vi "Find Safe Cell.vi"(0 "Cells":i32[](array[numeric]), 11 "error in (no error)":errorcluster) -> (4 "Safe Cells":i32[](array[numeric]), 6 "# of Safe Cells":i32, 15 "error out":errorcluster)   [LabVIEW 2014]
uses:
  Dragon Tamers.lvlib
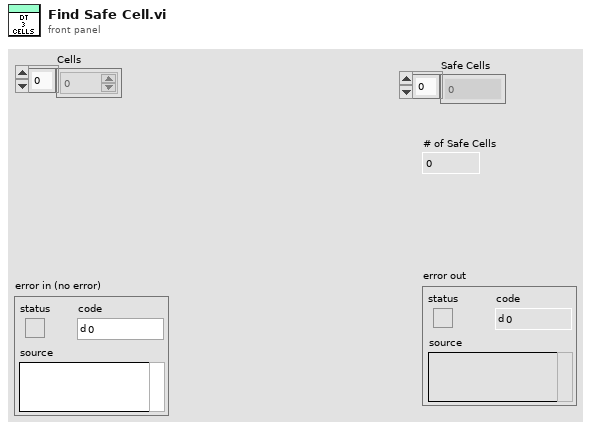
[diagram p1: front panel]
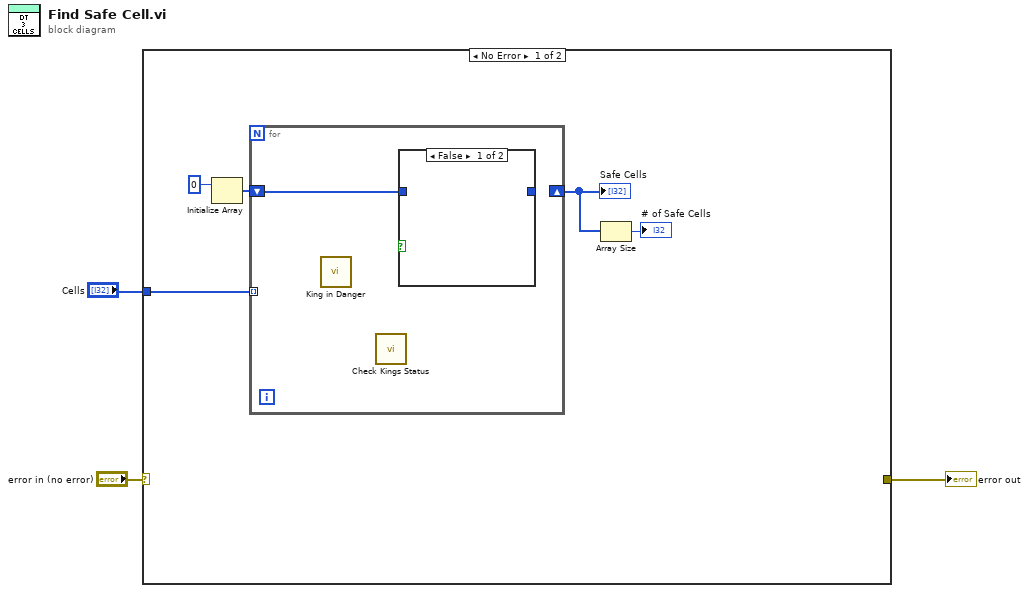
[diagram p0: block diagram]
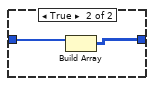
[diagram p2: hidden frame]
diagram:
  n1 = case shown="No Error" "error in (no error)" {
    selector: "error in (no error)" -> [_ w12]
    tunnel: [_ w12] -> w2
    tunnel: "Cells" -> [w8 _]
    frame No Error {
      n2 = Initialize Array(0) -> (w7:i32[])  [unwired: 1 in]
      n3 = for {
        tunnel: w8 -> [_] mode=indexing
        shift-right: [_] -> w5
        shift-left: w7 -> [w9]
        n4 = call "King in Danger.vi"() -> ()  [unwired: 13 in, 3 out]
        n5 = call "Check Kings Status.vi"() -> ()  [unwired: 11 in, 5 out]
        n6 = case shown="False" {
          selector: _ -> [_ _]
          tunnel: w9 -> [_ w11]
          tunnel: [_ w10] -> _
          frame False {
          }
          frame True {
            n7 = Build Array(w11) -> (w10:i32[][])  [unwired: 1 in]
          }
        }
      }
      "Safe Cells" <- w5
      n8 = Array Size(array=w5) -> (size(s)=→"# of Safe Cells":i32)
    }
    frame Error {
    }
  }
  "error out" <- w2
